vi "Set Fields.vi"(8 "error in":errorcluster, 10 "Fields":variant[](array[variant]), 11 "File Info in":refnum<class "File Info.lvclass">) -> (0 "error out":errorcluster, 3 "File Info out":refnum<class "File Info.lvclass">)   [LabVIEW 2019, in "Electronic Datasheet.lvlib" / "File Info.lvclass"]
uses:
  File Info.lvclass
  File Info.lvclass/File Info.ctl
  Electronic Datasheet.lvlib
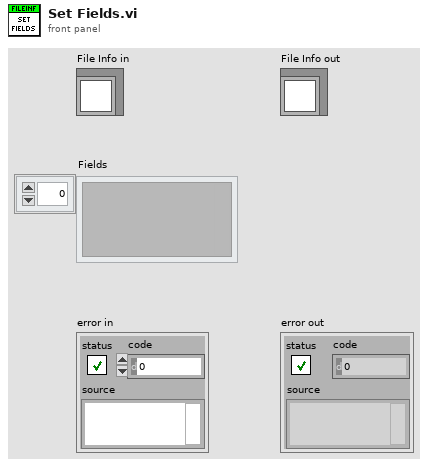
[diagram p1: front panel]
types:
  T1 = cluster{"FileName":string, "FileVersion":u8, "FileRevision":u8, "EDSVersion":string, "Description":string, "CreationTime":string, "CreationDate":string, "CreatedBy":string, "ModificationTime":string, "ModificationDate":string, "ModifiedBy":string}
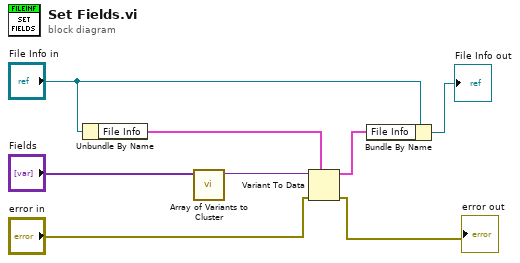
[diagram p0: block diagram]
diagram:
  n1 = Unbundle By Name("File Info in") -> ("File Info"=w4:T1)
  n2 = call "Array of Variants to Cluster.vi"("Fields"="Fields") -> ("Variant"=w6:variant)  [unwired: 10 in]
  n3 = Variant To Data(error in="error in", type=w4, Variant=w6) -> (data=w3:T1, error out=→"error out":errorcluster)
  n4 = Bundle By Name(cluster="File Info in", "File Info"=w3) -> (→"File Info out":refnum<class "File Info.lvclass">)
